vi "Sentran Accuracy Test DAA.vi"(8 "error in (no error)":errorcluster, 10 "Model in":refnum<class "Model.lvclass">, 11 "Test Actuator State in":refnum<class "Test Actuator State.lvclass">) -> (0 "error out":errorcluster, 1 "Pass":bool, 2 "Model out":refnum<class "Model.lvclass">, 3 "Test Actuator State out":refnum<class "Test Actuator State.lvclass">)   [LabVIEW 2016]
uses:
  Model/Model/Model.lvclass
  Typedefs/ActuatorSetPoints.ctl
  <vilib>/platform/TimedLoop/XDataNode/XDataNode.xnode
  <vilib>/Platform/TimedLoop/XDataNode/nitl_modes.ctl
  <vilib>/Platform/TimedLoop/XDataNode/XDNodeRunTimeDep.lvlib
  <vilib>/Platform/TimedLoop/XDataNode/wakeup.ctl
  <vilib>/Platform/TimedLoop/XDataNode/timing_clust.ctl
  Test Actuator State.lvclass
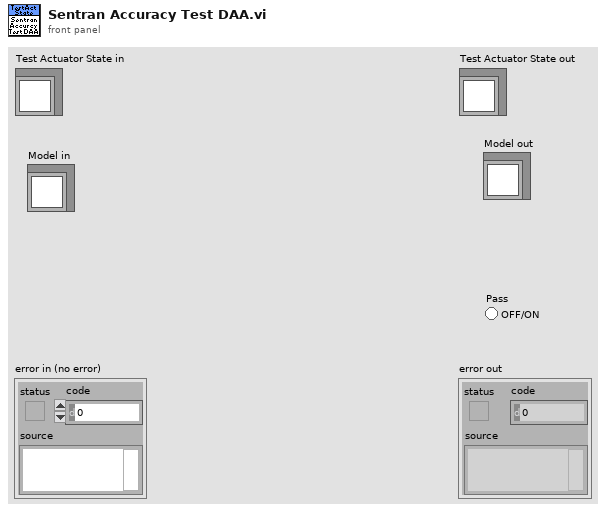
[diagram p1: front panel]
types:
  T1 = typedef "SentranAccuracyTestSettings.ctl" = cluster{"Force Tolerance (N)":dbl, "Force Modifies (%)":dbl[], "Process Time (s)":dbl, "Sample Time (s)":dbl, "Max Moment (NM)":dbl}
  T2 = typedef "FullForceScanSettings.ctl" = cluster{"Force Tolerance (N)":dbl, "DAA Force Set Points":T3[], "Process Time (s)":dbl, "Sample Time (s)":dbl, "Max Moment (NM)":dbl, "SAA Force Set Points":T3[]}
  T3 = typedef "ForcePair.ctl" = cluster{"Axial Force":dbl, "Lateral Force":dbl}
  T4 = typedef "ActuatorSetPoints.ctl" = cluster{"Axial Force":dbl, "Lateral Force":dbl, "FC1 Force":dbl, "FC2 Force":dbl}
  T5 = typedef "XDNodeRunTimeDep.lvlib/timing_clust.ctl" = cluster{"Expected End [f-1]":u64, "Actual End [f-1]":u64, "Finished Late? [f-1]":bool, "Expected End [i-1]":u64, "Actual End [i-1]":u64, "Finished Late? [i-1]":bool, "Expected Start [i]":u64, "Actual Start [i]":u64, "Expected Start [f]":u64, "Actual Start [f]":u64, "Source Name":string, "Structure Name":string, "Period":i64, "Deadline":i64, "Offset":i64, "Start":i64, "Priority":i32, "Timeout":i32, "Mode":T6, "Wakeup Reason":T7, "Error":errorcluster, "Source Type":string, "Secondary Source Type":string, "Global End Time":u64, "Global Start Time":u64, "Frame Duration":u64, "Iteration Duration":u64, "Assigned CPU":i32, "I/O Scan Engine Mode":u32}
  T6 = typedef "XDNodeRunTimeDep.lvlib/nitl_modes.ctl" = enum32{"No Change", "Process missed periods, maintain original phase", "Discard missed periods, maintain original phase", "Process missed periods, ignore original phase", "Discard missed periods, ignore original phase"}
  T7 = typedef "XDNodeRunTimeDep.lvlib/wakeup.ctl" = enum32{"Normal", "Aborted", "Asynchronous wakeup", "Timing source error", "Timed loop error", "Timeout"}
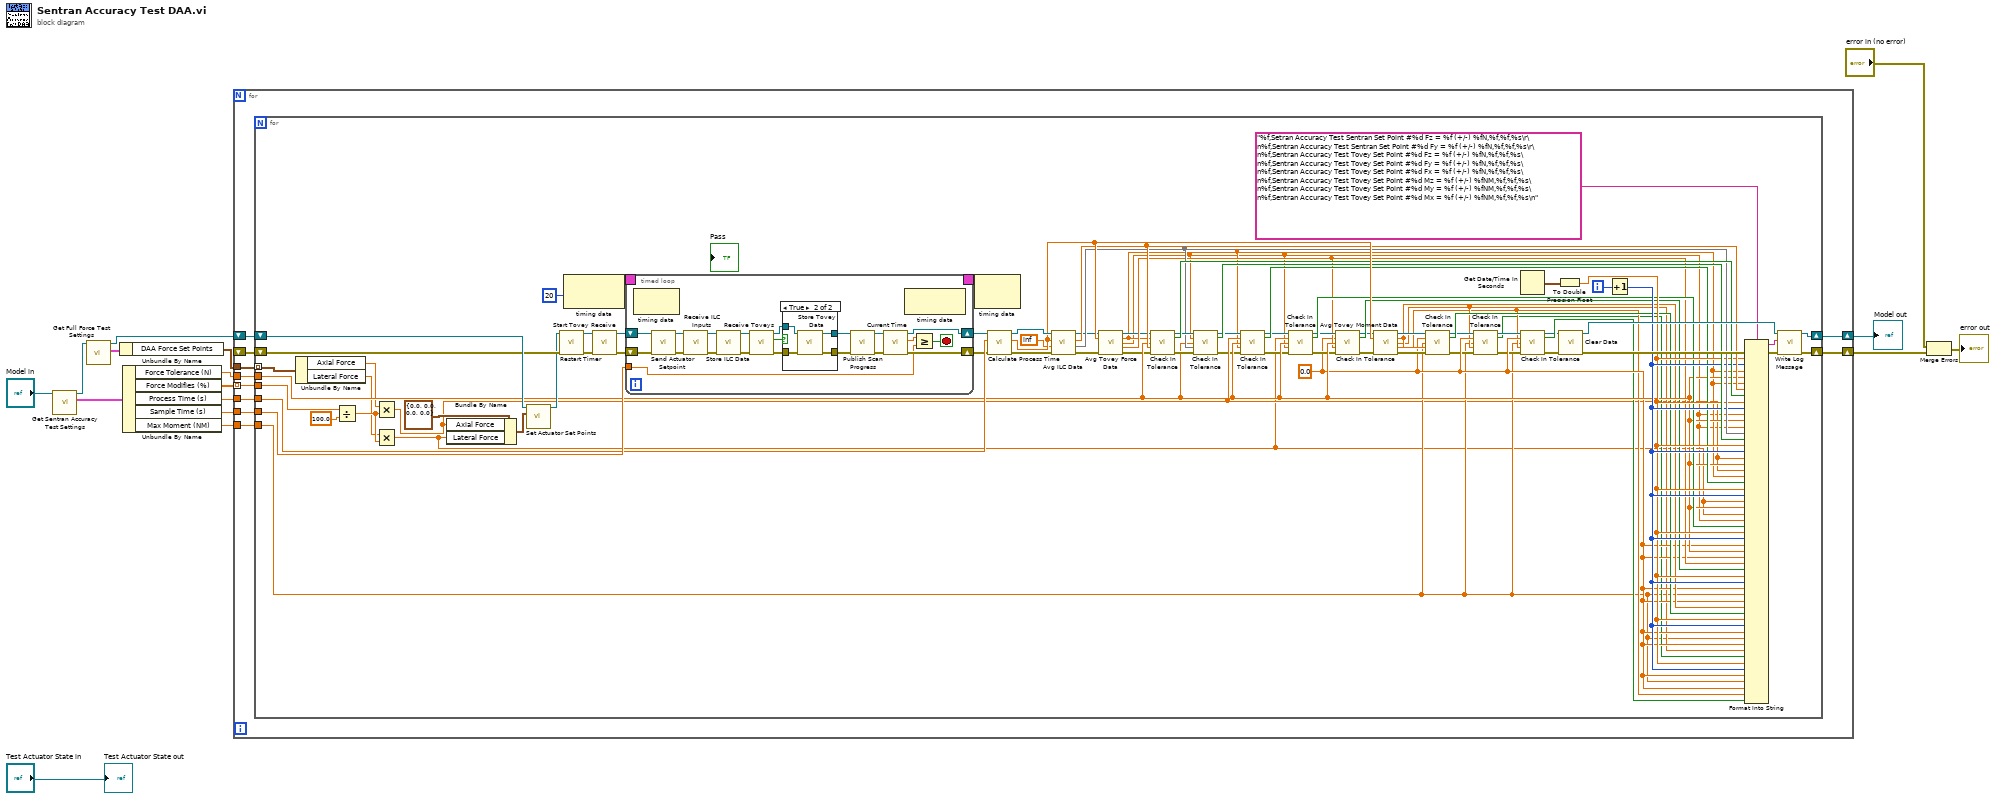
[diagram p0: block diagram]
diagram:
  n1 = call "Get Sentran Accuracy Test Settings.vi"("Model in"="Model in") -> ("Sentran Accuracy Test Settings"=w7:T1, "Model out"=w8:refnum<class "Model.lvclass">)  [unwired: 9 in]
  n2 = call "Get Full Force Test Settings.vi"("Model in"=w8) -> ("Full Force Test Settings"=w11:T2, "Model out"=w15:refnum<class "Model.lvclass">)  [unwired: 9 in]
  n3 = Unbundle By Name(w11) -> ("DAA Force Set Points"=w10:T3[])
  n4 = Unbundle By Name(w7) -> ("Force Tolerance (N)"=w4:dbl, "Force Modifies (%)"=w1:dbl[], "Process Time (s)"=w5:dbl, "Sample Time (s)"=w6:dbl, "Max Moment (NM)"=w3:dbl)
  n5 = for {
    tunnel: w10 -> [w23]
    tunnel: w6 -> [w22]
    tunnel: w5 -> [w21]
    tunnel: w4 -> [w20]
    tunnel: w3 -> [w19]
    shift-right: [w25] -> w13
    shift-left: w15 -> [w26]
    tunnel: w1 -> [w18] mode=indexing
    shift-right: [w24] -> w12
    shift-left: _ -> [w17]
    n6 = for {
      tunnel: w23 -> [w91] mode=indexing
      shift-right: [w101] -> w25
      shift-left: w26 -> [w105]
      tunnel: w22 -> [w104]
      tunnel: w21 -> [w86]
      tunnel: w20 -> [w68]
      shift-right: [w87] -> w24
      shift-left: w17 -> [w103]
      tunnel: w19 -> [w46]
      tunnel: w18 -> [w44]
      i -> [w98]
      w55 = 0.0
      n7 = Unbundle By Name(w91) -> ("Axial Force"=w41:dbl, "Lateral Force"=w39:dbl)
      n8 = Divide(x=w44, y=100.0) -> (x/y=w42:dbl)
      n9 = Multiply(x=w41, y=w42) -> (x*y=w40:dbl)
      n10 = Multiply(x=w39, y=w42) -> (x*y=w38:dbl)
      n11 = Bundle By Name(cluster=T4 {"Axial Force"=0.0, "Lateral Force"=0.0, "FC1 Force"=0.0, "FC2 Force"=0.0} ("Actuator Set Points"), "Axial Force"=w40, "Lateral Force"=w38) -> (w92:T4)
      n12 = call "Set Actuator Set Points.vi"("Actuator Set Points"=w92, "Model in"=w105) -> ("Model out"=w93:refnum<class "Model.lvclass">)  [unwired: 9 in]
      n13 = call "Restart Timer.vi"("error in (no error)"=w103, "Model in"=w93) -> ("error out"=w96:errorcluster, "Model out"=w97:refnum<class "Model.lvclass">)  [unwired: 8 in]
      n14 = node-c288(i64 20 ("Period")) -> (w29:T5)
      n15 = call "Start Tovey Receive.vi"("error in (no error)"=w96, "Model in"=w97) -> ("error out"=w94:errorcluster, "Model out"=w95:refnum<class "Model.lvclass">)  [unwired: 8 in]
      n16 = timed-loop {
        shift-right: [w120] -> w85
        shift-left: w95 -> [w126]
        shift-right: [w119] -> w83
        shift-left: w94 -> [w123]
        tunnel: w104 -> [w117]
        timing: w29 -> [_]
        timing-out: [_] -> w28
        stop <- w116 stop-if-true
        n17 = node-c288() -> ()  [unwired: 1 in, 1 out]
        n18 = call "Send Actuator Setpoint.vi"("error in (no error)"=w123, "Model in"=w126) -> ("error out"=w122:errorcluster, "Model out"=w125:refnum<class "Model.lvclass">)  [unwired: 8 in]
        n19 = call "Receive ILC Inputs.vi"("error in (no error)"=w122, "Model in"=w125) -> ("error out"=w121:errorcluster, "Model out"=w124:refnum<class "Model.lvclass">)  [unwired: 8 in]
        n20 = call "Store ILC Data.vi"("error in (no error)"=w121, "Model in"=w124) -> ("error out"=w114:errorcluster, "Model out"=w115:refnum<class "Model.lvclass">)  [unwired: 8 in]
        n21 = call "Receive Toveys.vi"("error in (no error)"=w114, "Model in"=w115) -> ("error out"=w112:errorcluster, "Data Received"=w111:bool, "Model out"=w113:refnum<class "Model.lvclass">)  [unwired: 7 in]
        n22 = case shown="True" w111 {
          tunnel: w113 -> [w130 w134]
          tunnel: w112 -> [w129 w133]
          tunnel: [w129 w132] -> w107
          tunnel: [w130 w131] -> w110
          frame False {
          }
          frame True {
            n23 = call "Store Tovey Data.vi"("error in (no error)"=w133, "Model in"=w134) -> ("error out"=w132:errorcluster, "Model out"=w131:refnum<class "Model.lvclass">)  [unwired: 8 in]
          }
        }
        n24 = call "Publish Scan Progress.vi"("error in (no error)"=w107, "Model in"=w110) -> ("error out"=w108:errorcluster, "Model out"=w109:refnum<class "Model.lvclass">)  [unwired: 8 in]
        n25 = call "Current Time.vi"("error in (no error)"=w108, "Model in"=w109) -> ("error out"=w119:errorcluster, "Time"=w118:dbl, "Model out"=w120:refnum<class "Model.lvclass">)  [unwired: 7 in]
        n26 = node-c288() -> ()  [unwired: 1 in, 1 out]
        n27 = Greater Or Equal?(x=w118, y=w117) -> (x >= y?=w116:bool)
      }
      n28 = node-c288(w28) -> ()  [unwired: 1 out]
      n29 = call "Calculate Process Time.vi"("error in (no error)"=w83, "Seconds"=w86, "Model in"=w85) -> ("error out"=w82:errorcluster, "Time"=w81:dbl, "Model out"=w84:refnum<class "Model.lvclass">)  [unwired: 6 in]
      n30 = call "Avg ILC Data.vi"("error in (no error)"=w82, "Before This Time"=inf, "After This Time"=w81, "Model in"=w84) -> ("error out"=w34:errorcluster, 1:w77, "Force"=w80:dbl, "Model out"=w37:refnum<class "Model.lvclass">)  [unwired: 4 in]
      n31 = call "Avg Tovey Force Data.vi"("Model in"=w37, "After This Time"=w81, "error in (no error)"=w34) -> ("Model out"=w36:refnum<class "Model.lvclass">, "Fz"=w31:dbl, "Fy"=w30:dbl, "Fx"=w59:dbl, "error out"=w33:errorcluster)  [unwired: 8 in]
      n32 = call "Check In Tolerance.vi"("Model in"=w36, "Expected"=w31, "Tolerance"=w68, "Actual"=w80, "error in (no error)"=w33) -> ("Model out"=w78:refnum<class "Model.lvclass">, "Pass"=w79:bool, "error out"=w75:errorcluster)  [unwired: 8 in]
      n33 = call "Check In Tolerance.vi"("Model in"=w78, "Expected"=w30, "Tolerance"=w68, "Actual"=w77, "error in (no error)"=w75) -> ("Model out"=w35:refnum<class "Model.lvclass">, "Pass"=w76:bool, "error out"=w32:errorcluster)  [unwired: 8 in]
      n34 = call "Check In Tolerance.vi"("Model in"=w35, "Expected"=w40, "Tolerance"=w68, "Actual"=w31, "error in (no error)"=w32) -> ("Model out"=w71:refnum<class "Model.lvclass">, "Pass"=w72:bool, "error out"=w65:errorcluster)  [unwired: 8 in]
      n35 = call "Check In Tolerance.vi"("Model in"=w71, "Expected"=w38, "Tolerance"=w68, "Actual"=w30, "error in (no error)"=w65) -> ("Model out"=w69:refnum<class "Model.lvclass">, "Pass"=w70:bool, "error out"=w64:errorcluster)  [unwired: 8 in]
      n36 = call "Check In Tolerance.vi"("Model in"=w69, "Expected"=w55, "Tolerance"=w68, "Actual"=w59, "error in (no error)"=w64) -> ("Model out"=w62:refnum<class "Model.lvclass">, "Pass"=w67:bool, "error out"=w63:errorcluster)  [unwired: 8 in]
      n37 = call "Avg Tovey Moment Data.vi"("Model in"=w62, "After This Time"=w81, "error in (no error)"=w63) -> ("Model out"=w61:refnum<class "Model.lvclass">, "Mz"=w58:dbl, "My"=w54:dbl, "Mx"=w53:dbl, "error out"=w60:errorcluster)  [unwired: 8 in]
      n38 = call "Check In Tolerance.vi"("Model in"=w61, "Expected"=w55, "Tolerance"=w46, "Actual"=w58, "error in (no error)"=w60) -> ("Model out"=w57:refnum<class "Model.lvclass">, "Pass"=w66:bool, "error out"=w49:errorcluster)  [unwired: 8 in]
      n39 = call "Check In Tolerance.vi"("Model in"=w57, "Expected"=w55, "Tolerance"=w46, "Actual"=w54, "error in (no error)"=w49) -> ("Model out"=w56:refnum<class "Model.lvclass">, "Pass"=w52:bool, "error out"=w48:errorcluster)  [unwired: 8 in]
      n40 = Get Date/Time In Seconds() -> (seconds since 1Jan1904=w99:timestamp)
      n41 = call "Check In Tolerance.vi"("Model in"=w56, "Expected"=w55, "Tolerance"=w46, "Actual"=w53, "error in (no error)"=w48) -> ("Model out"=w50:refnum<class "Model.lvclass">, "Pass"=w51:bool, "error out"=w47:errorcluster)  [unwired: 8 in]
      n42 = To Double Precision Float(number=w99) -> (double precision float=w73:dbl)
      n43 = call "Clear Data.vi"("error in (no error)"=w47, "Model in"=w50) -> ("error out"=w89:errorcluster, "Model out"=w102:refnum<class "Model.lvclass">)  [unwired: 8 in]
      n44 = Increment(x=w98) -> (x+1=w74:i32)
      n45 = Format Into String(format string="%f,Setran Accuracy Test Sentran Set Point #%d Fz = %f (+/-) %fN,%f,%f,%s\r\n%f,Sentran Accuracy Test Sentran Set Point #%d Fy = %f (+/-) %fN,%f,%f,%s\r\n%f,Sentran Accuracy Test Tovey Set Point #%d Fz = %f (+/-) %fN,%f,%f,%s\n%f,Sentran Accuracy Test Tovey Set Point #%d Fy = %f (+/-) %fN,%f,%f,%s\n%f,Sentran Accuracy Test Tovey Set Point #%d Fx = %f (+/-) %fN,%f,%f,%s\n%f,Sentran Accuracy Test Tovey Set Point #%d Mz = %f (+/-) %fNM,%f,%f,%s\n%f,Sentran Accuracy Test Tovey Set Point #%d My = %f (+/-) %fNM,%f,%f,%s\n%f,Sentran Accuracy Test Tovey Set Point #%d Mx = %f (+/-) %fNM,%f,%f,%s\n", error in=w89, w73, w74, w31, w68, w31, w80, w79, w73, w74, w30, w68, w30, w77, w76, w73, w74, w40, w68, w40, w31, w72, w73, w74, w38, w68, w38, w30, w70, w73, w74, w55, w68, w55, w59, w67, w73, w74, w55, w46, w55, w58, w66, w73, w74, w55, w46, w55, w54, w52, w73, w74, w55, w46, w55, w53, w51) -> (resulting string=w90:string, error out=w88:errorcluster)  [unwired: 1 in]
      n46 = call "Write Log Message.vi"("error in (no error)"=w88, "Message"=w90, "Model in"=w102) -> ("error out"=w87:errorcluster, "Model out"=w101:refnum<class "Model.lvclass">)  [unwired: 7 in]
    }
  }
  "Model out" <- w13
  n47 = Merge Errors("error in (no error)", w12) -> (→"error out":errorcluster)
  "Test Actuator State out" <- "Test Actuator State in"
